vi "In_S7F17.vi"(8 "error in (no error)":errorcluster, 11 "S7 Message Class in":refnum<class "S7 Message Class.lvclass">) -> (0 "error out":errorcluster, 1 "OK?":bool, 2 "PPID":string[](array[string]), 3 "S7 Message Class out":refnum<class "S7 Message Class.lvclass">)   [LabVIEW 2020, in "SECS Communication.lvlib" / "S7 Message Class.lvclass"]
uses:
  S7 Message Class.lvclass
  D:/Dropbox/SECS/SECS_GEM v1.0.6/Com/SECS Communication/SECS-II Class/SECS-II Class.lvclass
  SECS-II Class/SECS-II Class.lvclass/SECS-II Class.ctl
  SECS-II Class/Variant To Data_ASCII.vi
  SECS-II Class/SECS-II Class.lvclass
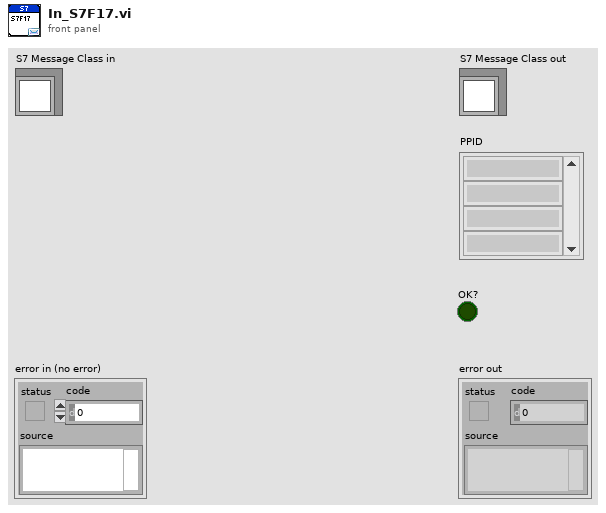
[diagram p1: front panel]
types:
  T1 = typedef "SECS Communication.lvlib/SECS-II Class.lvclass/Message Data.ctl" = cluster{"Index":i32, "Data Item Format":T2, "Format Code":T3, "Parent Index":i32, "Child Index":i32[], "Data":variant}
  T2 = typedef "SECS Communication.lvlib/SECS-II Class.lvclass/Data Item Format.ctl" = enum16{"Data Type", "Value"}
  T3 = typedef "SECS Communication.lvlib/SECS-II Class.lvclass/Format Code.ctl" = enum16{"L", "A", "B", "Boolean", "J", "I1", "I2", "I4", "I8", "U1", "U2", "U4", "U8", "F4", "F8", "Char"}
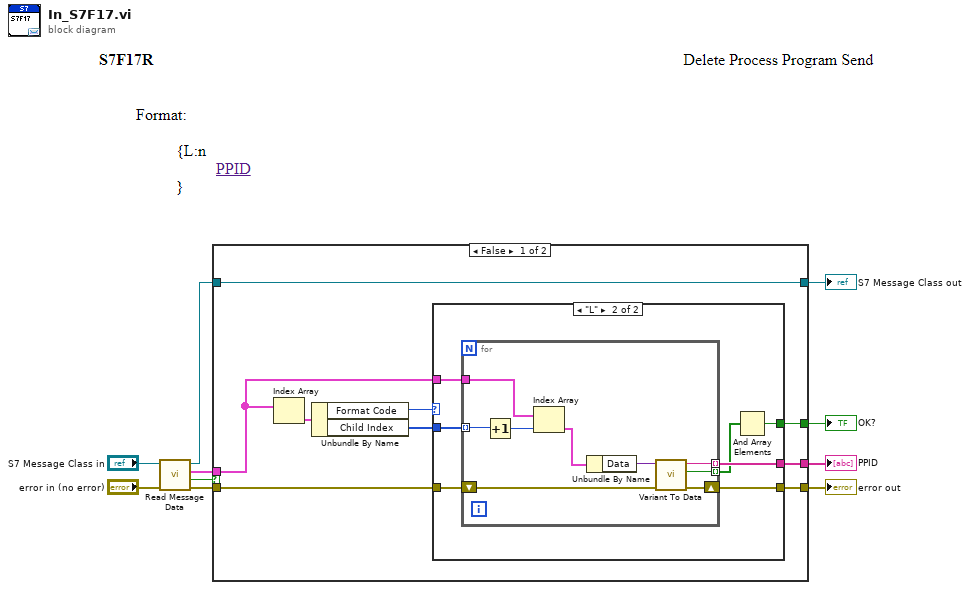
[diagram p0: block diagram]
diagram:
  n1 = call "Read Message Data.vi"("error in (no error)"="error in (no error)", "SECS-II Class in"="S7 Message Class in") -> ("error out"=w9:errorcluster, "Empty?"=w3:bool, "Message Data"=w10:T1[], "SECS-II Class out"=w2:refnum<class "S7 Message Class.lvclass">)  [unwired: 6 in]
  n2 = case shown="False" w3 {
    tunnel: w10 -> [w17 _]
    tunnel: w9 -> [w16 w37]
    tunnel: [w15 w37] -> w8
    tunnel: [w14 _] -> w5
    tunnel: [w12 _] -> w4
    tunnel: w2 -> [w11 w38]
    tunnel: [w11 w38] -> w1
    frame False {
      n3 = Index Array(array=w17) -> (element=w19:T1)  [unwired: 1 in]
      n4 = Unbundle By Name(w19) -> ("Format Code"=w13:T3, "Child Index"=w18:i32[])
      n5 = case shown="\"L\"" w13 {
        tunnel: w18 -> [_ w27]
        tunnel: w17 -> [_ w26]
        tunnel: w16 -> [w20 w25]
        tunnel: [w20 w24] -> w15
        tunnel: [_ w23] -> w14
        tunnel: [_ w21] -> w12
        frame Default {
        }
        frame "L" {
          n6 = for {
            tunnel: w27 -> [w35] mode=indexing
            tunnel: w26 -> [w36]
            shift-right: [w30] -> w24
            shift-left: w25 -> [w32]
            tunnel: [w29] -> w23 mode=indexing
            tunnel: [w28] -> w22 mode=indexing
            n7 = Increment(x=w35) -> (x+1=w34:i32)
            n8 = Index Array(array=w36, index=w34) -> (element=w33:T1)
            n9 = Unbundle By Name(w33) -> ("Data"=w31:variant)
            n10 = call-poly "Variant To Data.vi"("error in (no error)"=w32, "Variant"=w31) -> ("error out"=w30:errorcluster, "OK?"=w28:bool, "Data"=w29:string)  [unwired: 7 in]
          }
          n11 = And Array Elements(Boolean array=w22) -> (logical AND=w21:bool)
        }
      }
    }
    frame True {
    }
  }
  "error out" <- w8
  "S7 Message Class out" <- w1
  "PPID" <- w5
  "OK?" <- w4
